vi "Read Marker (Power Marker).vi"(0 "VISA resource name":refnum<visa-resource-name>, 5 "Marker Type (0:Marker)":i32(ring) items=["Marker", "Reference Marker", "Delta", "All"], 11 "error in (no error)":errorcluster) -> (4 "VISA resource name out":refnum<visa-resource-name>, 6 "Power Density Cluster":T1 {"Density Delta" format="%.3f"; "Power Delta" format="%.3f"; "Density Reference" format="%.3f"; "Power Reference" format="%.3f"; "Density Marker" format="%.3f"; "Power Marker" format="%.3f"}, 15 "error out":errorcluster)   [LabVIEW 2023, in "Anritsu Signal Analyzer Series.lvlib"]
doc: "Reads the Power Marker data."
uses:
  Anritsu Signal Analyzer Series.lvlib
panel:
  # "dBm"
  # "dBm"
  # "dBm"
  # "dBm"
  # "dB"
  # "dB"
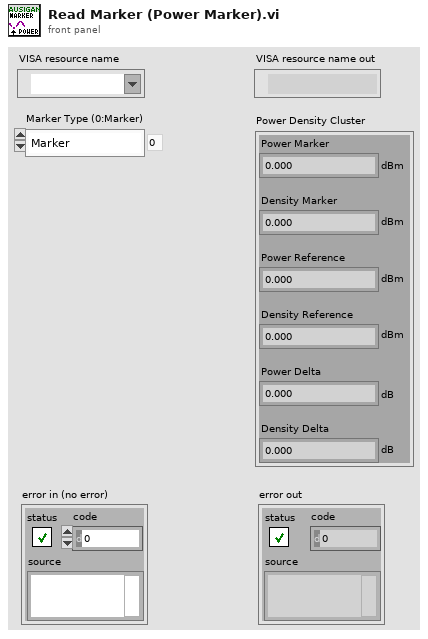
[diagram p1: front panel]
types:
  T1 = cluster{"Power Marker":dbl, "Density Marker":dbl, "Power Reference":dbl, "Density Reference":dbl, "Power Delta":dbl, "Density Delta":dbl}
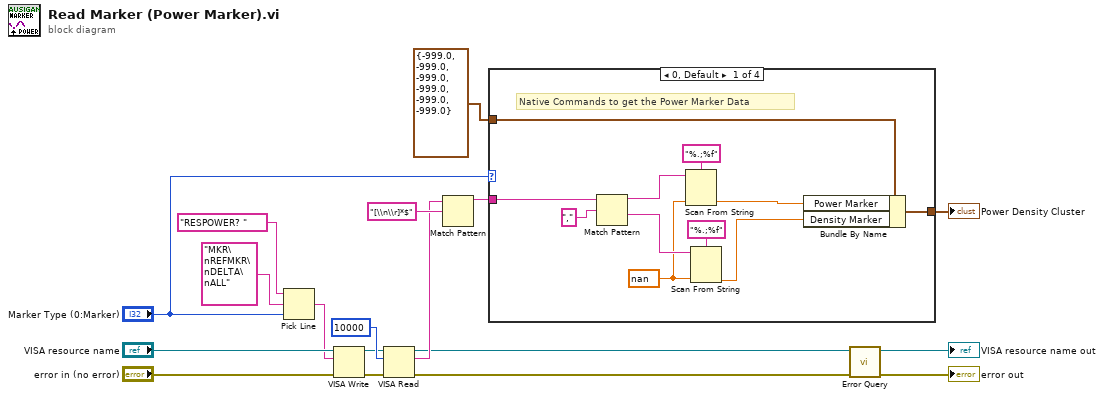
[diagram p0: block diagram]
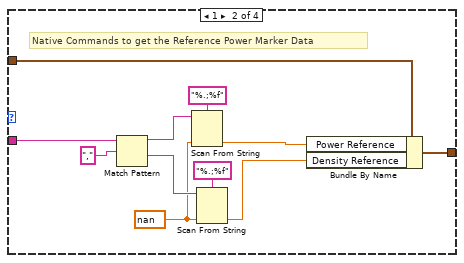
[diagram p2: hidden frame]
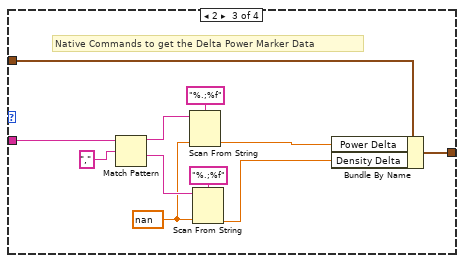
[diagram p3: hidden frame]
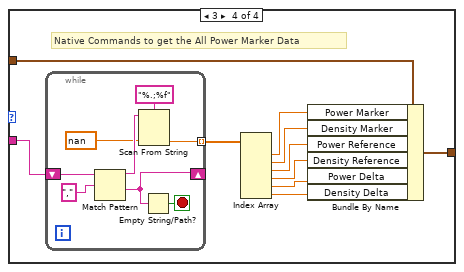
[diagram p4: hidden frame]
diagram:
  n1 = Pick Line(string ("")="RESPOWER? " ("_Command"), multi-line string="MKR\nREFMKR\nDELTA\nALL" ("文字列"), line index="Marker Type (0:Marker)") -> (output string=w2:string)
  n2 = VISA Write(VISA resource name="VISA resource name", write buffer=w2, error in (no error)="error in (no error)") -> (VISA resource name out=w11:refnum<visa-resource-name>, error out=w12:errorcluster)  [unwired: 1 out]
  n3 = VISA Read(VISA resource name=w11, byte count=u32 10000 ("byte count (0)"), error in (no error)=w12) -> (VISA resource name out=w5:refnum<visa-resource-name>, read buffer=w7:string, error out=w6:errorcluster)  [unwired: 1 out]
  n4 = Match Pattern(string=w7, regular expression="[\\n\\r]*$") -> (before substring=w9:string)  [unwired: 1 in, 3 out]
  n5 = case shown="0, Default" "Marker Type (0:Marker)" {
    tunnel: w9 -> [w25 w36 w47 w60]
    tunnel: T1 {"Power Marker"=-999.0, "Density Marker"=-999.0, "Power Reference"=-999.0, "Density Reference"=-999.0, "Power Delta"=-999.0, "Density Delta"=-999.0} ("Frequency or Time and Level Cluster") -> [w22 w33 w44 w61]
    tunnel: [w19 w30 w41 w52] -> w15
    frame 0, Default {
      w23 = nan ("_Default")
      # "Native Commands to get the Power Marker Data"
      n6 = Match Pattern(string=w25, regular expression=",") -> (before substring=w27:string, after substring=w24:string)  [unwired: 1 in, 2 out]
      n7 = Scan From String(format string="%.;%f" ("Format String"), input string=w27, default 1=w23) -> (output 1=w21:dbl)  [unwired: 2 in, 3 out]
      n8 = Scan From String(format string="%.;%f" ("Format String"), input string=w24, default 1=w23) -> (output 1=w20:dbl)  [unwired: 2 in, 3 out]
      n9 = Bundle By Name(cluster=w22, "Power Marker"=w21, "Density Marker"=w20) -> (w19:T1)
    }
    frame 1 {
      w34 = nan ("_Default")
      # "Native Commands to get the Reference Power Marker Data"
      n10 = Match Pattern(string=w36, regular expression=",") -> (before substring=w38:string, after substring=w35:string)  [unwired: 1 in, 2 out]
      n11 = Scan From String(format string="%.;%f" ("Format String"), input string=w38, default 1=w34) -> (output 1=w32:dbl)  [unwired: 2 in, 3 out]
      n12 = Scan From String(format string="%.;%f" ("Format String"), input string=w35, default 1=w34) -> (output 1=w31:dbl)  [unwired: 2 in, 3 out]
      n13 = Bundle By Name(cluster=w33, "Power Reference"=w32, "Density Reference"=w31) -> (w30:T1)
    }
    frame 2 {
      w45 = nan ("_Default")
      # "Native Commands to get the Delta Power Marker Data"
      n14 = Match Pattern(string=w47, regular expression=",") -> (before substring=w49:string, after substring=w46:string)  [unwired: 1 in, 2 out]
      n15 = Scan From String(format string="%.;%f" ("Format String"), input string=w49, default 1=w45) -> (output 1=w43:dbl)  [unwired: 2 in, 3 out]
      n16 = Scan From String(format string="%.;%f" ("Format String"), input string=w46, default 1=w45) -> (output 1=w42:dbl)  [unwired: 2 in, 3 out]
      n17 = Bundle By Name(cluster=w44, "Power Delta"=w43, "Density Delta"=w42) -> (w41:T1)
    }
    frame 3 {
      # "Native Commands to get the All Power Marker Data"
      n18 = while {
        shift-right: [w63] -> _
        shift-left: w60 -> [w65]
        tunnel: [w62] -> w59 mode=indexing
        stop <- w64 stop-if-true
        n19 = Match Pattern(string=w65, regular expression=",") -> (before substring=w67:string, after substring=w63:string)  [unwired: 1 in, 2 out]
        n20 = Scan From String(format string="%.;%f" ("Format String"), input string=w67, default 1=nan ("_Default")) -> (output 1=w62:dbl)  [unwired: 2 in, 3 out]
        n21 = Empty String/Path?(string/path=w63) -> (empty?=w64:bool)
      }
      n22 = Index Array(array=w59) -> (element #1=w53:dbl, element #2=w54:dbl, element #3=w55:dbl, element #4=w56:dbl, element #5=w57:dbl, element #6=w58:dbl)  [unwired: 6 in]
      n23 = Bundle By Name(cluster=w61, "Power Marker"=w53, "Density Marker"=w54, "Power Reference"=w55, "Density Reference"=w56, "Power Delta"=w57, "Density Delta"=w58) -> (w52:T1)
    }
  }
  "Power Density Cluster" <- w15
  n24 = call "Error Query.vi"("error in (no error)"=w6, "VISA resource name"=w5) -> ("error out"=→"error out":errorcluster, "VISA resource name out"=→"VISA resource name out":refnum<visa-resource-name>)  [unwired: 6 in, 2 out]
